vi "GetNameOfVI.vi"(10 "NameOfVi2Call(optional)":string, 11 "VIIn":refnum<vi>) -> (3 "Name":string)   [LabVIEW 2021, in "YActor.lvclass"]
uses:
  YActor.lvclass
  YActor.lvclass/YActor.ctl
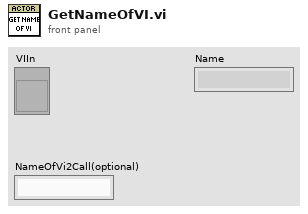
[diagram p1: front panel]
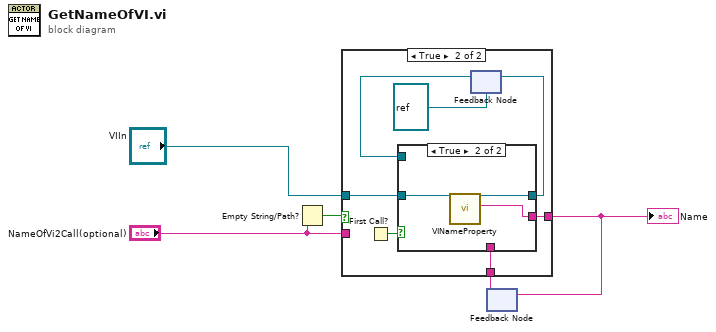
[diagram p0: block diagram]
diagram:
  n1 = Empty String/Path?(string/path="NameOfVi2Call(optional)") -> (empty?=w5:bool)
  n2 = feedback #1() -> (w1:string)  [unwired: 1 in]
  n3 = case shown="True" w5 {
    tunnel: w1 -> [_ w11]
    tunnel: [w6 w10] -> w3
    tunnel: "VIIn" -> [_ w9]
    tunnel: "NameOfVi2Call(optional)" -> [w6 _]
    frame False {
    }
    frame True {
      n4 = First Call?() -> (First Call?: T/F=w7:bool)
      n5 = feedback #2(refnum<vi> refnum ("Cmd VI ref")) -> (w8:refnum<vi>)
      n6 = case shown="True" w7 {
        tunnel: w9 -> [_ w18]
        tunnel: [w15 w17] -> w10
        tunnel: w11 -> [w15 _]
        tunnel: [w14 w16] -> w12
        tunnel: w8 -> [w14 _]
        frame False {
        }
        frame True {
          n7 = call "VINameProperty.vi"("VIIn"=w18) -> ("Name"=w17:string, "VIOut"=w16:refnum<vi>)  [unwired: 9 in]
        }
      }
      n8 = feedback-in #2(w12) -> ()
    }
  }
  "Name" <- w3
  n9 = feedback-in #1(w3) -> ()
